vi "Discretization_DiscretizeR.vi"(6 "dT_Seconds":dbl, 9 "ContR":T1, 11 "Outputs":i32) -> (3 "DiscR":T1)   [LabVIEW 2019, in "Trajectory_Library.lvlib"]
doc: "Creates a new LINEAR SYSTEM data cluster with the specified values. \n\n\nInputs: \n - XXX -- XXX.\n\nOutputs:\n - XXX -- XXX."
uses:
  <vilib>/Analysis/Matrix/Datatypes/RealMatrix.ctl
  Trajectory_Library.lvlib
  <vilib>/Analysis/Matrix/NI_Matrix.lvlib
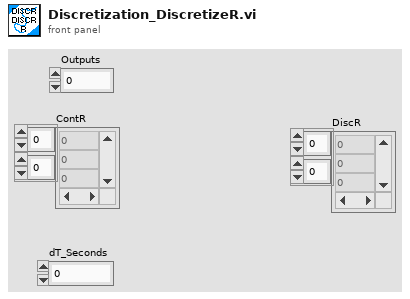
[diagram p1: front panel]
types:
  T1 = typedef "NI_Matrix.lvlib/RealMatrix.ctl" = dbl[][]
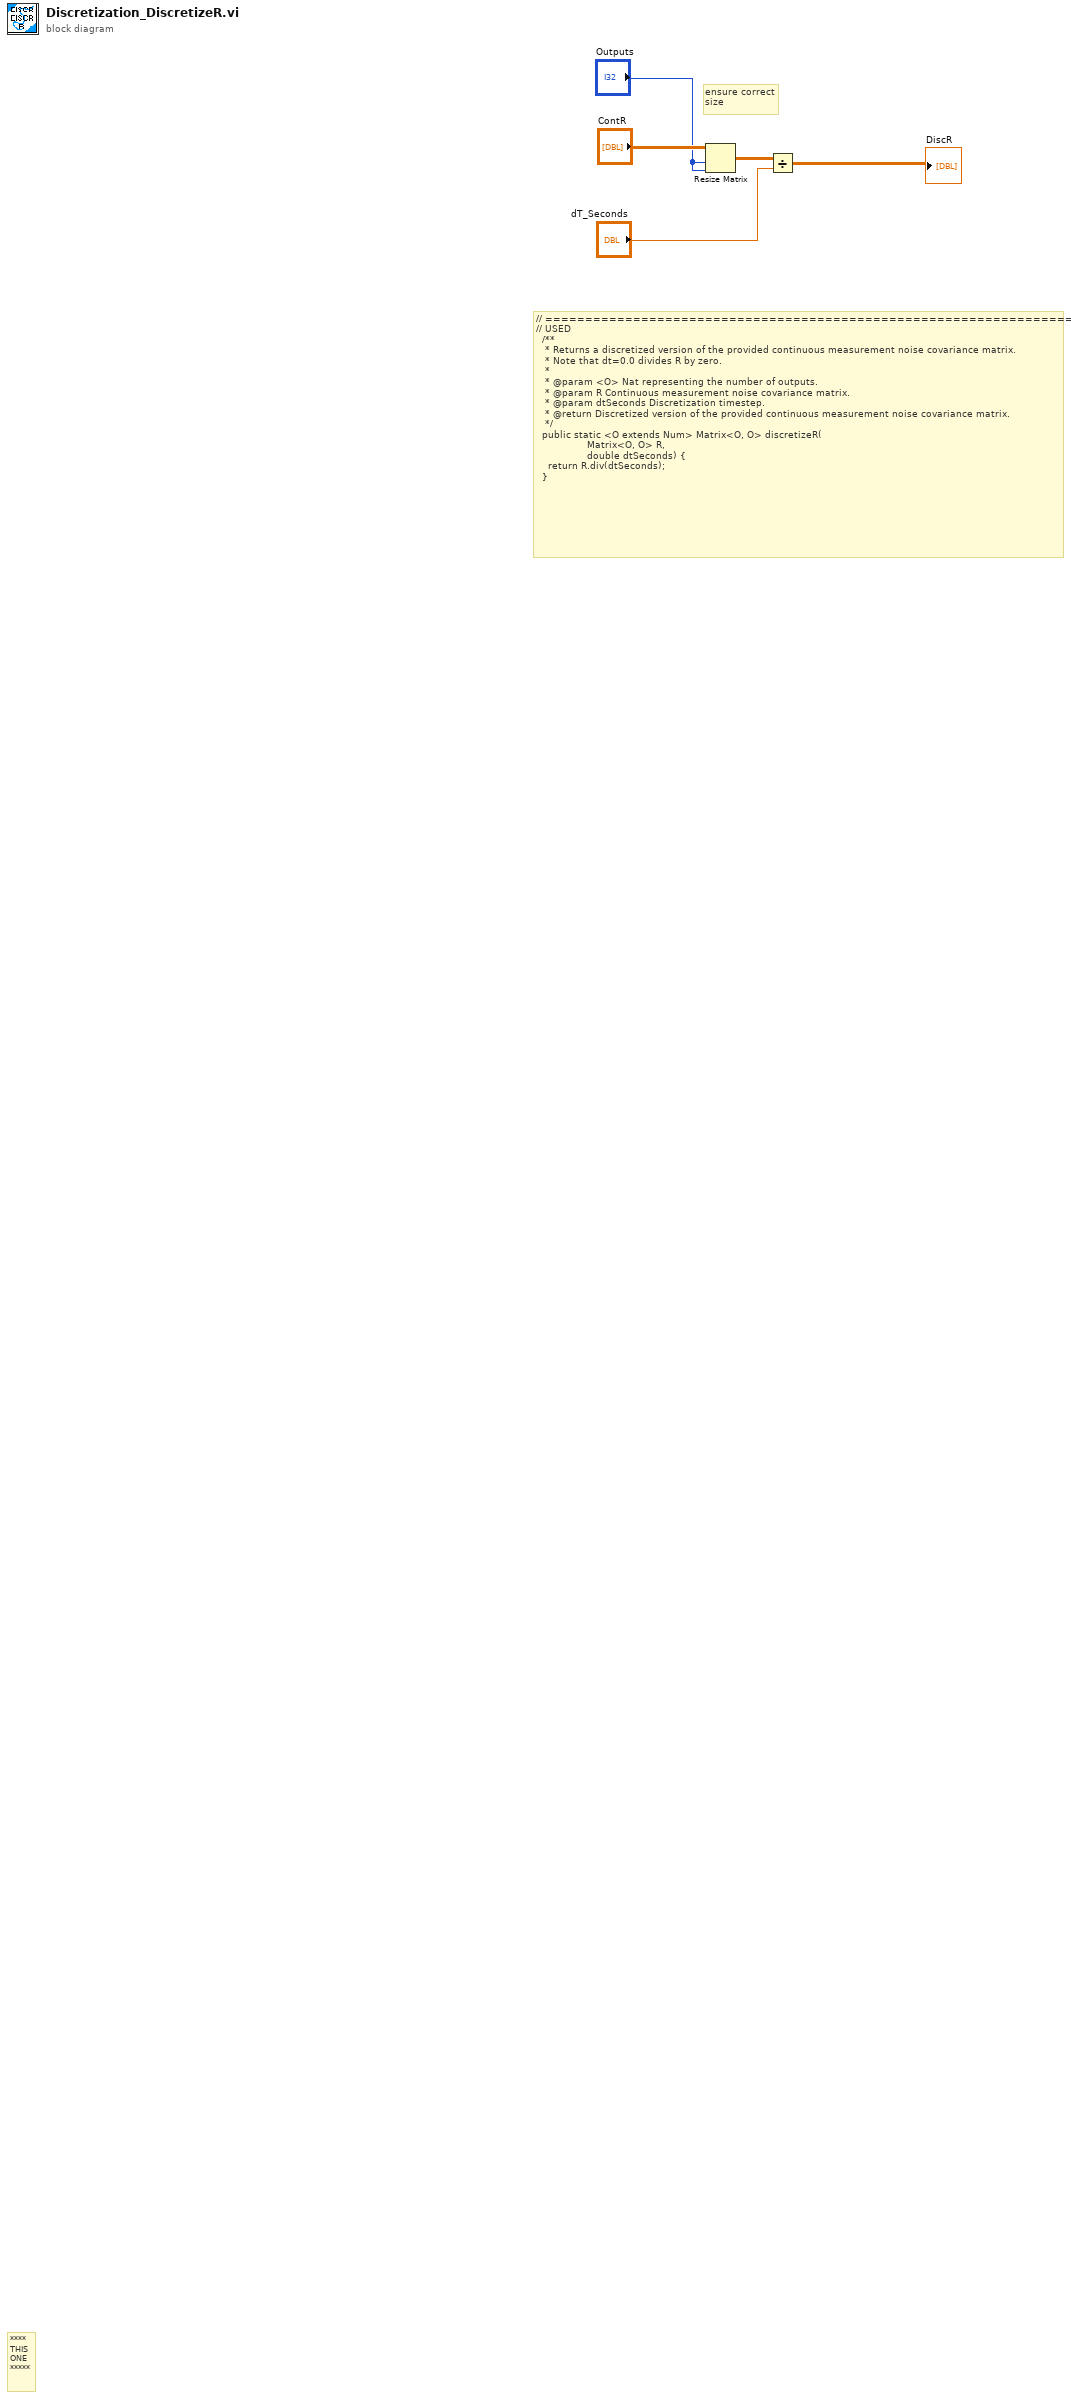
[diagram p0: block diagram]
diagram:
  # "// ==================================================================\n// USED\n  /**\n   * Returns a discretized version of the provided continuous measurement noise covariance matrix.\n   * Note that dt=0.0 divides R by zero.\n   *\n   * @param <O> Nat representing the number of outputs.\n   * @param R Continuous measurement noise covariance matrix.\n   * @param dtSeconds Discretization timestep.\n   * @return Discretized version of the provided continuous measurement noise covariance matrix.\n   */\n  public static <O extends Num> Matrix<O, O> discretizeR(\n                 Matrix<O, O> R, \n                 double dtSeconds) {\n    return R.div(dtSeconds);\n  }"
  # "ensure correct\nsize"
  # "****\nTHIS\nONE\n*****"
  n1 = Resize Matrix(1:"Outputs", 2:"Outputs", 4:"ContR") -> (0:w3:T1)
  n2 = Divide(x=w3, y="dT_Seconds") -> (x/y=→"DiscR":T1)
